vi "3_ReadDatatoWaveform.vi"(0 "file path (IN)":path, 11 "error in (no error)":errorcluster) -> (1 "Ch 1 Data":dbl[](array[numeric]), 2 "Ch 2 Data":dbl[](array[numeric]), 3 "t0":dbl, 4 "file path (OUT)":path, 6 "Waveform Graph":waveform(dbl)[](graph), 12 "Ch 3 Data":dbl[](array[numeric]), 13 "Ch 4 Data":dbl[](array[numeric]), 14 "dt":dbl, 15 "error out":errorcluster)   [LabVIEW 2020]
uses:
  <vilib>/Utility/file.llb/Read Delimited Spreadsheet (string).vi
  <vilib>/Utility/file.llb/Read Delimited Spreadsheet (DBL).vi
panel:
  out "Spread Sheet Display":string[][](array[string])
  out "Data Display":dbl[][](array[numeric])
  # "Channel 1"
  # "Channel 2"
  # "Channel 4"
  # "Channel 3"
  # "C:\\Users\\zbmbdt\\Desktop\\Assignment\\2022\\LabVIEW Project\\ACModule_TRR\\TRR_sourcewaveform\\tempTRRgraphdata.csv"
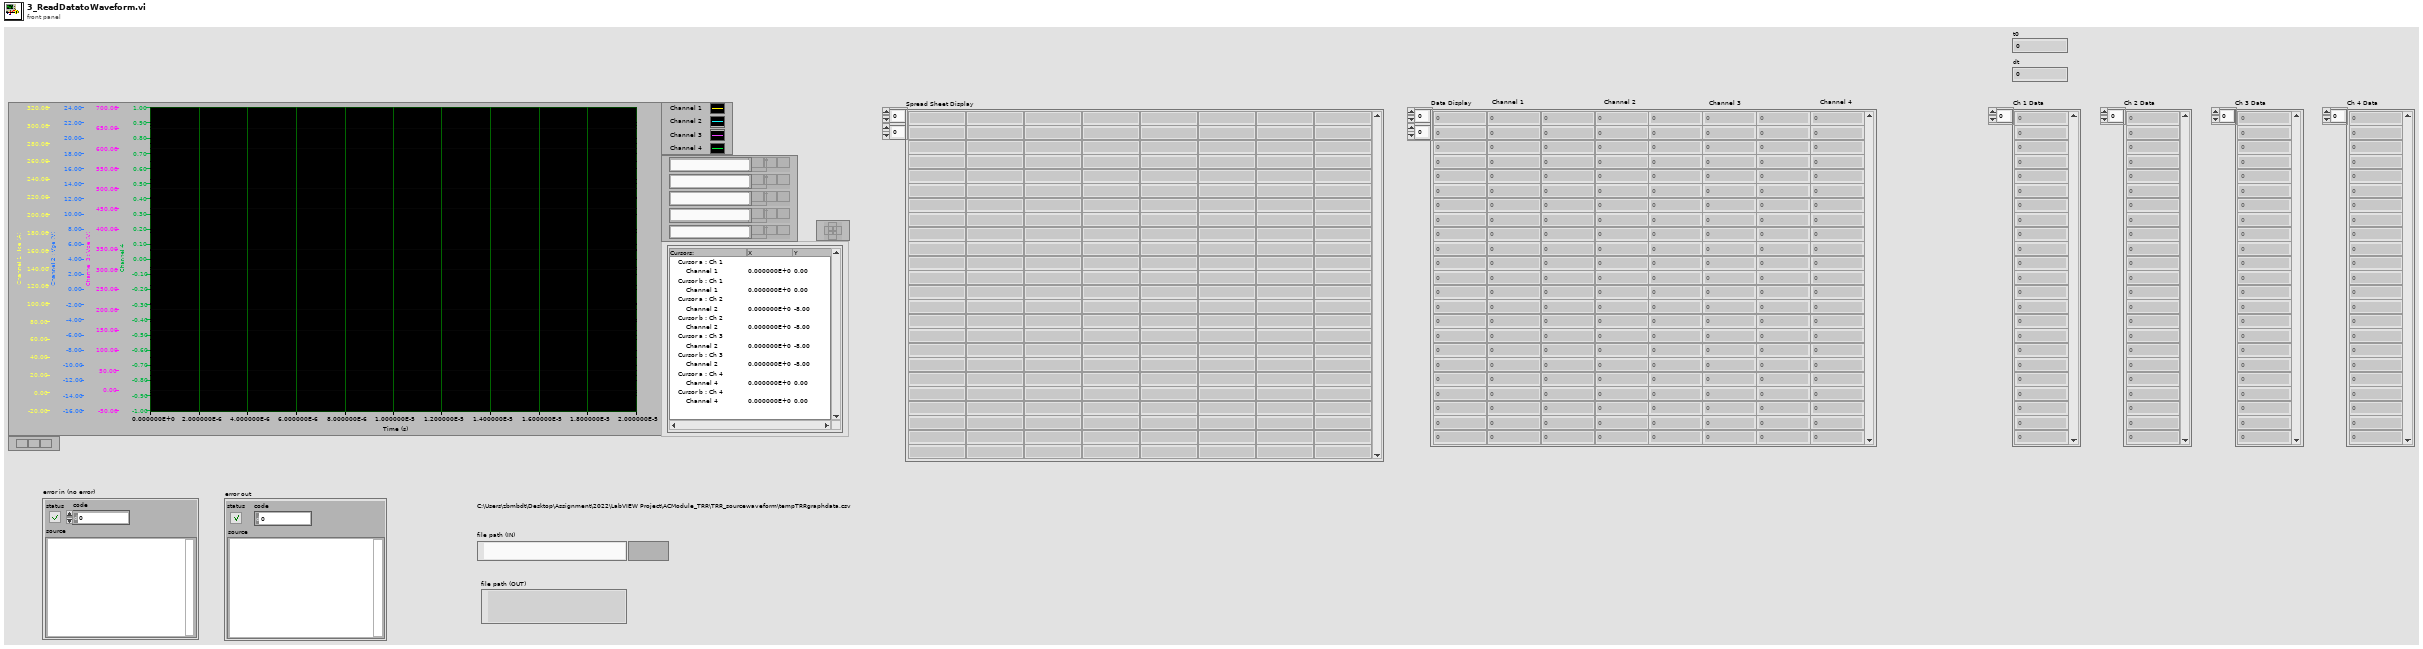
[diagram p1: front panel]
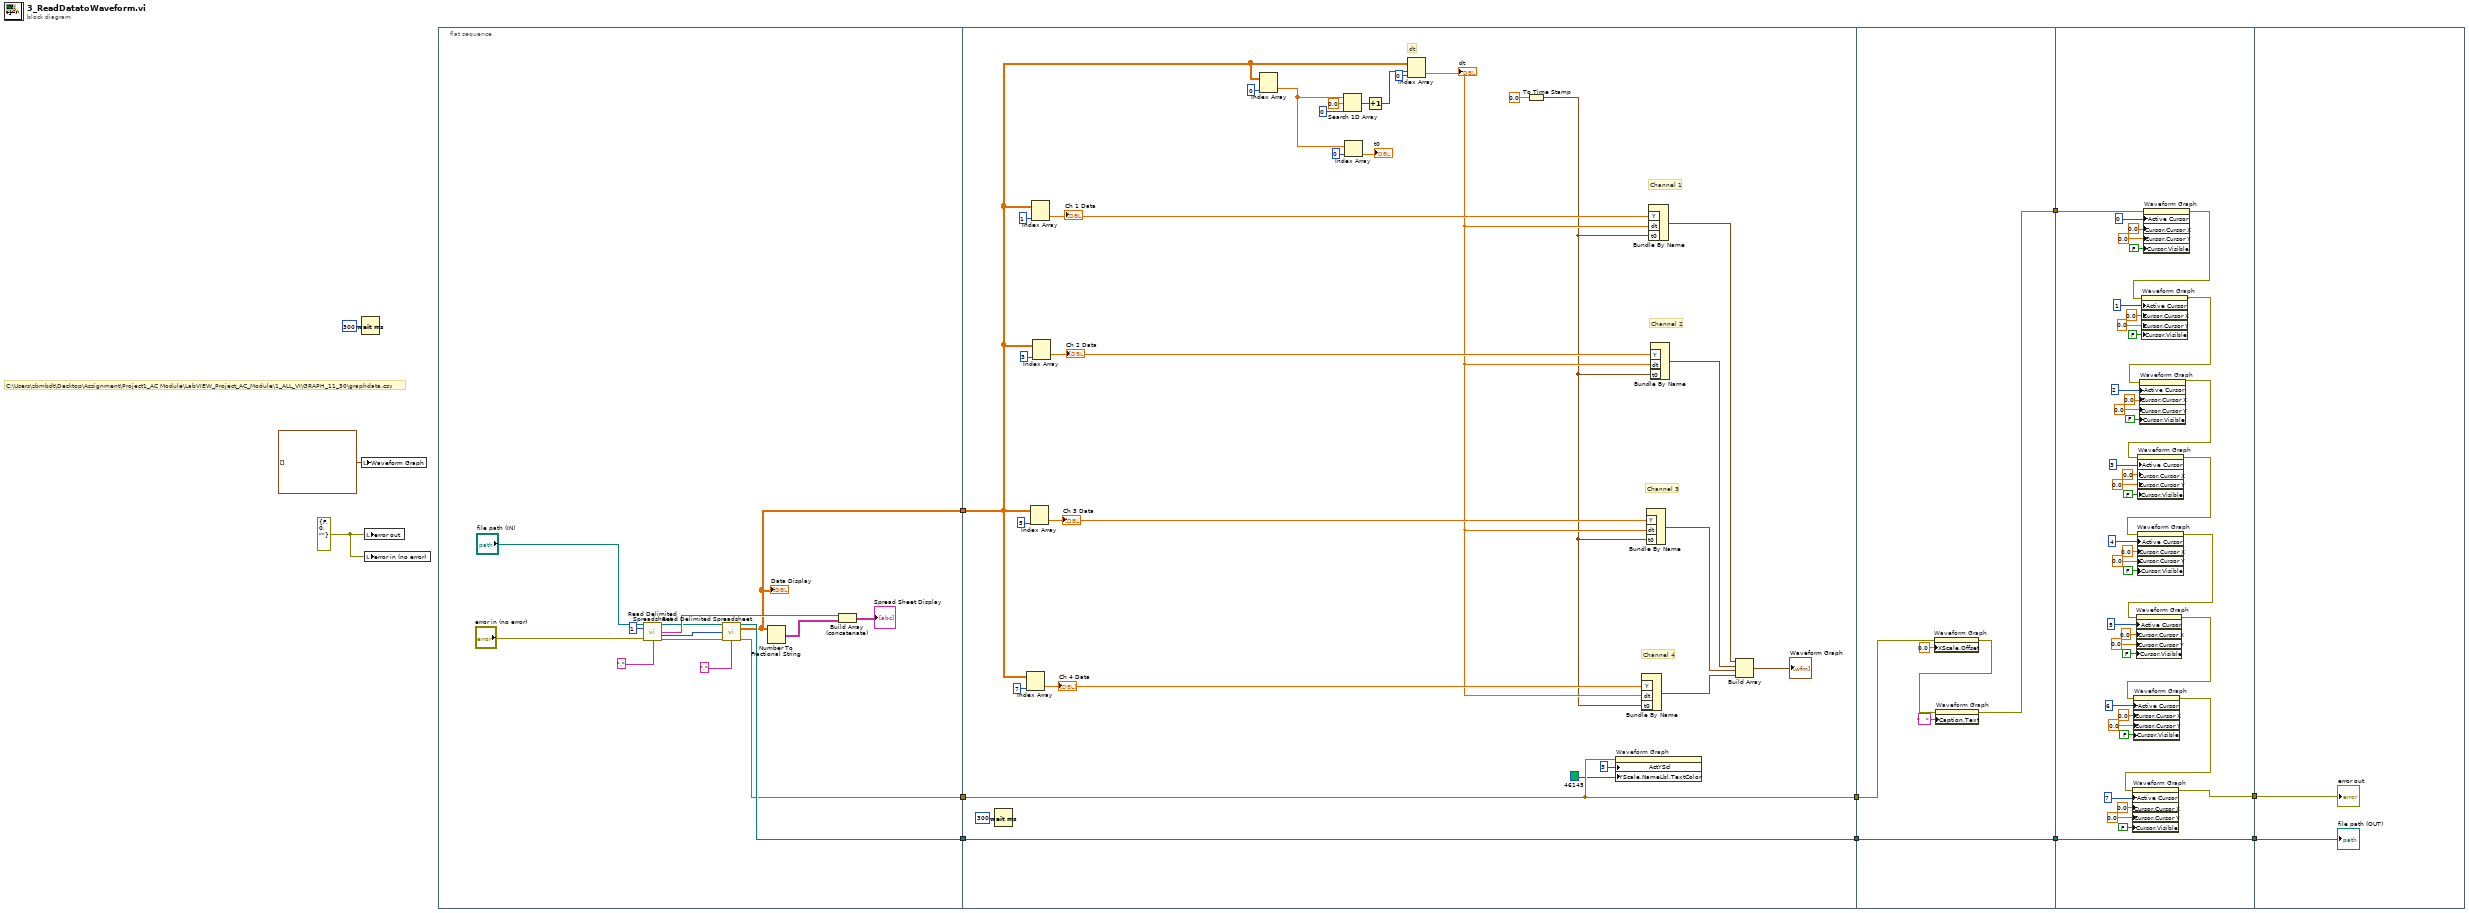
[diagram p0: block diagram]
diagram:
  w2 = errorcluster {"status"=FALSE, "code"=0, "source"=""} ("error out")
  # "C:\\Users\\zbmbdt\\Desktop\\Assignment\\Project1_AC Module\\LabVIEW_Project_AC_Module\\1_ALL_VI\\GRAPH_11_30\\graphdata.csv"
  n1 = Wait (ms)(milliseconds to wait=u32 300) -> ()  [unwired: 1 out]
  n2 = local write "Waveform Graph"(waveform(dbl)[] [] ("Waveform Graph")) -> ()
  n3 = local write "error out"(w2) -> ()
  n4 = local write "error in (no error)"(w2) -> ()
  n5 = flat-sequence {
    tunnel: [w14] -> w7
    tunnel: [w13] -> w6
    tunnel: [w15] -> w5
    tunnel: [w29] -> w12
    tunnel: [w52] -> w11
    tunnel: w7 -> [w32]
    tunnel: w6 -> [w29]
    tunnel: w5 -> [w52]
    tunnel: w12 -> [w62]
    tunnel: w11 -> [w63]
    tunnel: [w63] -> w10
    tunnel: [w59] -> w9
    tunnel: w10 -> [w105]
    tunnel: [w105] -> w4
    tunnel: w9 -> [w104]
    tunnel: [w64] -> w3
    tunnel: w4 -> [w107]
    tunnel: w3 -> [w106]
    frame #0 {
      n6 = call-poly <vilib>:"Read Delimited Spreadsheet.vi"("file path (dialog if empty)"="file path (IN)", "number of rows (all:-1)"=1, "error in (no error)"="error in (no error)", "delimiter (\\t)"="," ("delimiter (\\t)")) -> ("new file path (Not A Path if cancelled)"=w20:path, "first row"=w21:string[], "mark after read (chars.)"=w19:i32, "error out"=w25:errorcluster)  [unwired: 6 in, 2 out]
      n7 = call-poly <vilib>:"Read Delimited Spreadsheet.vi"("file path (dialog if empty)"=w20, "start of read offset (chars.:0)"=w19, "error in (no error)"=w25, "delimiter (\\t)"="," ("delimiter (\\t)")) -> ("new file path (Not A Path if cancelled)"=w15:path, "all rows"=w14:dbl[][], "error out"=w13:errorcluster)  [unwired: 6 in, 3 out]
      "Data Display" <- w14
      n8 = Number To Fractional String(number=w14) -> (F-format string=w22:string[][])  [unwired: 3 in]
      n9 = Build Array (concatenate)(w21, w22) -> (→"Spread Sheet Display":string[][])
    }
    frame #1 {
      # "Channel 4"
      # "Channel 2"
      # "dt"
      # "Channel 3"
      # "Channel 1"
      n10 = Wait (ms)(milliseconds to wait=u32 300) -> ()  [unwired: 1 out]
      n11 = Index Array(array=w32, index (col)=7 ("disabled index (col)")) -> (element=w35:dbl[])  [unwired: 1 in]
      "Ch 4 Data" <- w35
      n12 = Index Array(array=w32, index (col)=5 ("disabled index (col)")) -> (element=w54:dbl[])  [unwired: 1 in]
      "Ch 3 Data" <- w54
      n13 = Index Array(array=w32, index (col)=1 ("disabled index (col)")) -> (element=w42:dbl[])  [unwired: 1 in]
      "Ch 1 Data" <- w42
      n14 = Index Array(array=w32, index (col)=3 ("disabled index (col)")) -> (element=w38:dbl[])  [unwired: 1 in]
      "Ch 2 Data" <- w38
      n15 = Index Array(array=w32, index (col)=0 ("disabled index (col)")) -> (element=w41:dbl[])  [unwired: 1 in]
      n16 = Search 1D Array(1D array=w41, element=0.0, start index (0)=0) -> (index of element=w46:i32)
      n17 = Index Array(array=w41, index=0) -> (element=→"t0":dbl)
      n18 = Increment(x=w46) -> (x+1=w44:i32)
      n19 = Index Array(array=w32, index (row)=w44, index (col)=0 ("disabled index (col)")) -> (element=w31:dbl)
      "dt" <- w31
      n20 = To Time Stamp(1:0.0 ("number")) -> (0:w30:timestamp)
      n21 = property on="Waveform Graph" class="WFGraph (strict)"(error in=w29, "ActYScl"=3 ("Active Y Scale"), "YScale.NameLbl.TextColor"=u32 46145 ("Y Scale.Name Label.Text Colors:Text Color")) -> ()  [unwired: 1 in, 2 out]
      n22 = Bundle By Name("Y"=w35, "dt"=w31, "t0"=w30) -> (w33:waveform(dbl))  [unwired: 1 in]
      n23 = Bundle By Name("Y"=w54, "dt"=w31, "t0"=w30) -> (w49:waveform(dbl))  [unwired: 1 in]
      n24 = Bundle By Name("Y"=w42, "dt"=w31, "t0"=w30) -> (w55:waveform(dbl))  [unwired: 1 in]
      n25 = Bundle By Name("Y"=w38, "dt"=w31, "t0"=w30) -> (w36:waveform(dbl))  [unwired: 1 in]
      n26 = Build Array(w55, w36, w49, w33) -> (→"Waveform Graph":waveform(dbl)[])
    }
    frame #2 {
      n27 = property on="Waveform Graph" class="WFGraph (strict)"(error in=w62, "XScale.Offset"=0.0 ("X Scale.Offset and Multiplier:Offset")) -> (error out=w60:errorcluster)  [unwired: 1 in, 1 out]
      n28 = property on="Waveform Graph" class="WFGraph (strict)"(error in=w60, "Caption.Text"="   ") -> (error out=w59:errorcluster)  [unwired: 1 in, 1 out]
    }
    frame #3 {
      n29 = property on="Waveform Graph" class="WFGraph (strict)"(error in=w104, "Active Cursor"=u32 0, "Cursor.Cursor X"=0.0 ("Cursor.Cursor Position:Cursor X"), "Cursor.Cursor Y"=0.0 ("Cursor.Cursor Position:Cursor Y"), "Cursor.Visible"=FALSE) -> (error out=w71:errorcluster)  [unwired: 1 in, 1 out]
      n30 = property on="Waveform Graph" class="WFGraph (strict)"(error in=w71, "Active Cursor"=u32 1, "Cursor.Cursor X"=0.0 ("Cursor.Cursor Position:Cursor X"), "Cursor.Cursor Y"=0.0 ("Cursor.Cursor Position:Cursor Y"), "Cursor.Visible"=FALSE) -> (error out=w70:errorcluster)  [unwired: 1 in, 1 out]
      n31 = property on="Waveform Graph" class="WFGraph (strict)"(error in=w70, "Active Cursor"=u32 2, "Cursor.Cursor X"=0.0 ("Cursor.Cursor Position:Cursor X"), "Cursor.Cursor Y"=0.0 ("Cursor.Cursor Position:Cursor Y"), "Cursor.Visible"=FALSE) -> (error out=w69:errorcluster)  [unwired: 1 in, 1 out]
      n32 = property on="Waveform Graph" class="WFGraph (strict)"(error in=w69, "Active Cursor"=u32 3, "Cursor.Cursor X"=0.0 ("Cursor.Cursor Position:Cursor X"), "Cursor.Cursor Y"=0.0 ("Cursor.Cursor Position:Cursor Y"), "Cursor.Visible"=FALSE) -> (error out=w68:errorcluster)  [unwired: 1 in, 1 out]
      n33 = property on="Waveform Graph" class="WFGraph (strict)"(error in=w68, "Active Cursor"=u32 4, "Cursor.Cursor X"=0.0 ("Cursor.Cursor Position:Cursor X"), "Cursor.Cursor Y"=0.0 ("Cursor.Cursor Position:Cursor Y"), "Cursor.Visible"=FALSE) -> (error out=w67:errorcluster)  [unwired: 1 in, 1 out]
      n34 = property on="Waveform Graph" class="WFGraph (strict)"(error in=w67, "Active Cursor"=u32 5, "Cursor.Cursor X"=0.0 ("Cursor.Cursor Position:Cursor X"), "Cursor.Cursor Y"=0.0 ("Cursor.Cursor Position:Cursor Y"), "Cursor.Visible"=FALSE) -> (error out=w66:errorcluster)  [unwired: 1 in, 1 out]
      n35 = property on="Waveform Graph" class="WFGraph (strict)"(error in=w66, "Active Cursor"=u32 6, "Cursor.Cursor X"=0.0 ("Cursor.Cursor Position:Cursor X"), "Cursor.Cursor Y"=0.0 ("Cursor.Cursor Position:Cursor Y"), "Cursor.Visible"=FALSE) -> (error out=w65:errorcluster)  [unwired: 1 in, 1 out]
      n36 = property on="Waveform Graph" class="WFGraph (strict)"(error in=w65, "Active Cursor"=u32 7, "Cursor.Cursor X"=0.0 ("Cursor.Cursor Position:Cursor X"), "Cursor.Cursor Y"=0.0 ("Cursor.Cursor Position:Cursor Y"), "Cursor.Visible"=FALSE) -> (error out=w64:errorcluster)  [unwired: 1 in, 1 out]
    }
    frame #4 {
      "error out" <- w106
      "file path (OUT)" <- w107
    }
  }
